vi "Bot.vi"(7 "BotData":T4, 10 "MatchState":T1, 11 "GameState":T2) -> (0 "error out":errorcluster, 3 "Move":T5)   [LabVIEW 2015, in "RandomBot.lvlib"]
uses:
  RandomBot.lvlib
  TronVIEWBotAPI/MovementDirection.ctl
  TronVIEWBotAPI/BotData.ctl
  TronVIEWBotAPI/GameState.ctl
  TronviewGame/Board/Position.ctl
  TronVIEWBotAPI/MatchState.ctl
  <vilib>/Analysis/1siggen.llb/Riffle Array (I32).vi
  TronVIEWGameUtilities/TronVIEWGameUtilities.lvlib
  TronVIEWBotAPI/TronVIEWBotAPI.lvlib
  <vilib>/Analysis/NI_AALBase.lvlib
  TronviewGame/Board/Board.lvclass
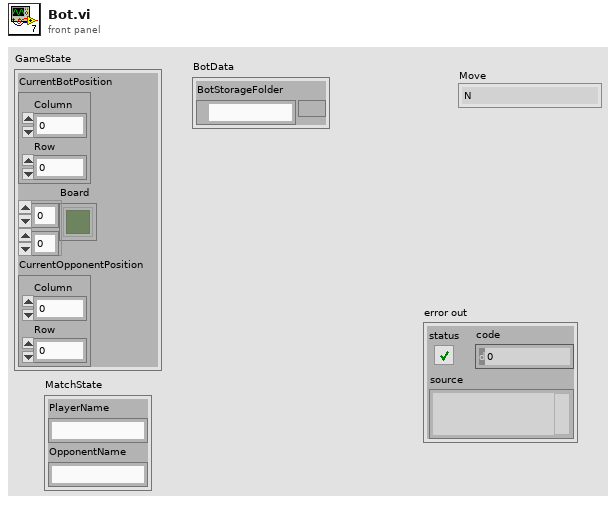
[diagram p1: front panel]
types:
  T1 = typedef "TronVIEWBotAPI.lvlib/MatchState.ctl" = cluster{"PlayerName":string, "OpponentName":string}
  T2 = typedef "TronVIEWBotAPI.lvlib/GameState.ctl" = cluster{"CurrentBotPosition":T3, "Board":bool[][], "CurrentOpponentPosition":T3}
  T3 = typedef "TronviewGame.lvlib/Board.lvclass/Position.ctl" = cluster{"Column":i32, "Row":i32}
  T4 = typedef "TronVIEWBotAPI.lvlib/BotData.ctl" = cluster{"BotStorageFolder":path}
  T5 = typedef "TronVIEWBotAPI.lvlib/MovementDirection.ctl" = enum16{"N", "S", "W", "E"}
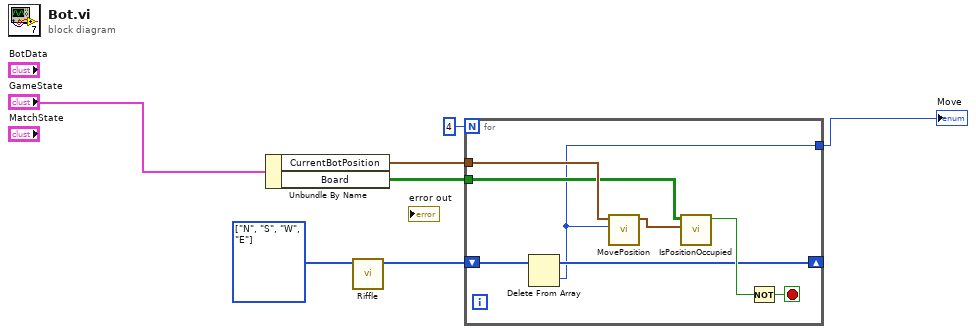
[diagram p0: block diagram]
diagram:
  w4 = T5[] [enum."N", enum."S", enum."W", enum."E"] items=["N", "S", "W", "E"]
  n1 = Unbundle By Name("GameState") -> ("CurrentBotPosition"=w7:T3, "Board"=w6:bool[][])
  n2 = call-poly <vilib>:"Riffle.vi"("X"=w4) -> ("Riffled {X}"=w3:i32[])  [unwired: 8 in, 2 out]
  n3 = for {
    N: 4 -> [_]
    tunnel: w7 -> [w15]
    tunnel: w6 -> [w13]
    shift-right: [w9] -> _
    shift-left: w3 -> [w10]
    tunnel: [w8] -> w2
    stop <- w11 stop-if-true
    n4 = Delete From Array(array=w10) -> (deleted portion=w8:i32, array with subset deleted=w9:i32[])  [unwired: 2 in]
    n5 = call "MovePosition.vi"("Direction"=w8, "PlayerPosition"=w15) -> ("NewPlayerPosition"=w14:T3)  [unwired: 9 in]
    n6 = call "IsPositionOccupied.vi"("Position"=w14, "Board"=w13) -> ("Occupied?"=w12:bool)  [unwired: 9 in]
    n7 = Not(x=w12) -> (.not. x?=w11:bool)
  }
  "Move" <- w2
